vi "Write Cylinder1.vi"(10 "IActuatorCylinder.lvclass":refnum<class "IActuatorCylinder.lvclass">, 11 "SingleCylinderActuator in":refnum<class "SingleCylinderActuator.lvclass">) -> (3 "SingleCylinderActuator out":refnum<class "SingleCylinderActuator.lvclass">)   [LabVIEW 2015, in "SingleCylinderActuator.lvclass"]
uses:
  SingleCylinderActuator.lvclass
  ActuatorCylinder/IActuatorCylinder/IActuatorCylinder.lvclass
  SingleCylinderActuator.lvclass/SingleCylinderActuator.ctl
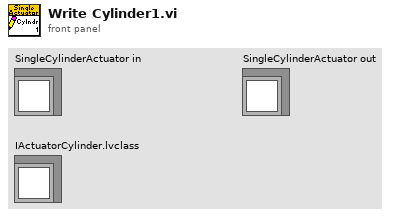
[diagram p1: front panel]
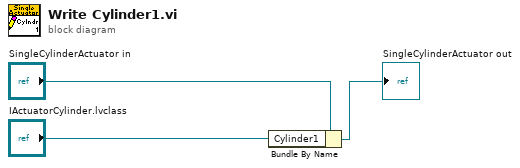
[diagram p0: block diagram]
diagram:
  n1 = Bundle By Name(cluster="SingleCylinderActuator in", "Cylinder1"="IActuatorCylinder.lvclass") -> (→"SingleCylinderActuator out":refnum<class "SingleCylinderActuator.lvclass">)
